vi "Write Cmd.vi"(8 "error in":errorcluster, 10 "CmdStruct":T1, 11 "CPC in":refnum<class "CPC.lvclass">) -> (0 "error out":errorcluster, 2 "Buffer":string, 3 "CPC out":refnum<class "CPC.lvclass">)   [LabVIEW 2014, in "CPC.lvclass"]
uses:
  CPC.lvclass
  <vilib>/Instr/_visa.llb/VISA Flush IO Buffer Mask.ctl
  Controls/CmdStruct.ctl
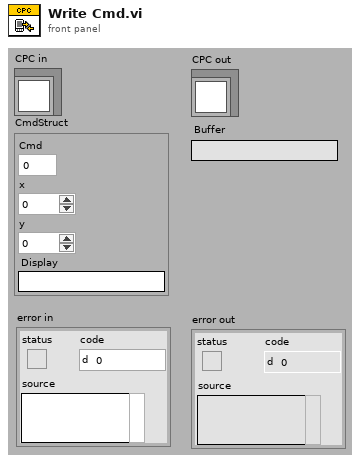
[diagram p1: front panel]
types:
  T1 = typedef "CmdStruct.ctl" = cluster{"Cmd":u8, "x":i64, "y":i64, "Display":string}
  T2 = typedef "VISA Flush IO Buffer Mask.ctl" = u16
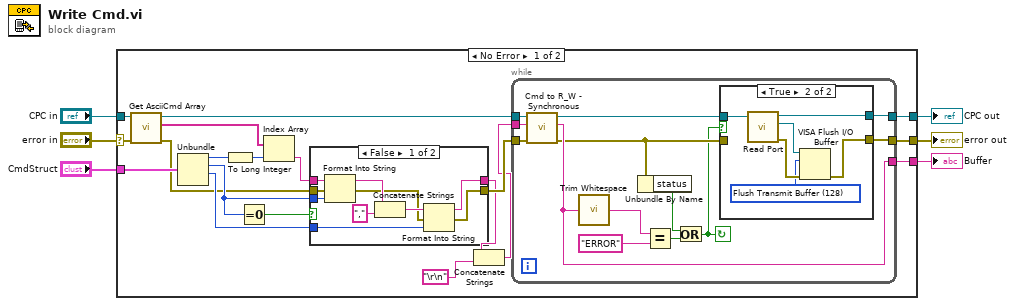
[diagram p0: block diagram]
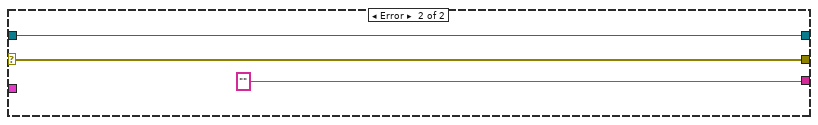
[diagram p4: hidden frame]
diagram:
  n1 = case shown="No Error" "error in" {
    selector: "error in" -> [w24 w61]
    tunnel: [w20 w61] -> w5
    tunnel: [w21 w60] -> w3
    tunnel: "CPC in" -> [w25 w60]
    tunnel: "CmdStruct" -> [w23 _]
    tunnel: [w22 ""] -> w1
    frame No Error {
      n2 = call-dynamic "Get AsciiCmd Array.vi"("error in"=w24, "CPC in"=w25) -> ("error out"=w11:errorcluster, "AsciiCmd"=w18:string[], "CPC out"=w19:refnum<class "CPC.lvclass">)  [unwired: 7 in]
      n3 = Unbundle(w23) -> ("Cmd"=w17:u8, "x"=w13:i64, "y"=w12:i64)  [unwired: 1 out]
      n4 = To Long Integer(number=w17) -> (32bit integer=w16:i32)
      n5 = Equal To 0?(x=w13) -> (x = 0?=w15:bool)
      n6 = Index Array(array=w18, index=w16) -> (element=w14:string)
      n7 = case shown="False" w15 {
        tunnel: w14 -> [w55 w58]
        tunnel: [w50 w58] -> w8
        tunnel: w13 -> [w56 _]
        tunnel: w12 -> [w51 _]
        tunnel: w11 -> [w49 w57]
        tunnel: [w47 w57] -> w10
        frame False {
          n8 = Format Into String(initial string=w55, error in=w49, w56) -> (resulting string=w54:string, error out=w48:errorcluster)  [unwired: 1 in]
          n9 = Concatenate Strings(w54, "," ("string")) -> (w52:string)
          n10 = Format Into String(initial string=w52, error in=w48, w51) -> (resulting string=w50:string, error out=w47:errorcluster)  [unwired: 1 in]
        }
        frame True {
        }
      }
      n11 = Concatenate Strings(w8, "\r\n") -> (w7:string)
      n12 = while {
        tunnel: [w34] -> w22
        tunnel: [w28] -> w21
        tunnel: [w27] -> w20
        tunnel: w19 -> [w38]
        tunnel: w7 -> [w37]
        tunnel: w10 -> [w36]
        stop <- w26 continue-if-true
        n13 = call-dynamic "Cmd to R_W - Synchronous.vi"("error in"=w36, "write buffer"=w37, "Serial IO in"=w38) -> ("error out"=w29:errorcluster, "read buffer"=w34:string, "Serial IO out"=w30:refnum<class "CPC.lvclass">)  [unwired: 6 in]
        n14 = call <vilib>:"Trim Whitespace.vi"("string"=w34) -> ("trimmed string"=w33:string)  [unwired: 1 in]
        n15 = Unbundle By Name(w29) -> ("status"=w31:bool)
        n16 = Equal?(x=w33, y="ERROR") -> (x = y?=w32:bool)
        n17 = Or(x=w31, y=w32) -> (x .or. y?=w26:bool)
        n18 = case shown="True" w26 {
          tunnel: w30 -> [w40 w46]
          tunnel: w29 -> [w39 _]
          tunnel: [w40 w45] -> w28
          tunnel: [w39 w42] -> w27
          frame False {
          }
          frame True {
            w43 = T2 128 items=["Flush Receive Buffer"=16, "Write Transmit Buffer to Device"=32, "Flush Receive Buffer (No I/O)"=64, "Flush Transmit Buffer"=128] ("Mask")
            n19 = call "Read Port.vi"("Serial IO in"=w46) -> ("error out"=w44:errorcluster, "Port"=w41:refnum<visa-resource-name>, "Serial IO out"=w45:refnum<class "CPC.lvclass">)  [unwired: 8 in]
            n20 = VISA Flush I/O Buffer(VISA resource name=w41, mask (16)=w43, error in (no error)=w44) -> (error out=w42:errorcluster)  [unwired: 1 out]
          }
        }
      }
    }
    frame Error {
    }
  }
  "error out" <- w5
  "CPC out" <- w3
  "Buffer" <- w1
